vi "Test TCC Request Chamber State Returns Heater State.vi"(8 "error in (no error)":errorcluster, 11 "Thermal Chamber Controller Test In":refnum<class "Thermal Chamber Controller Test.lvclass">) -> (0 "error out":errorcluster, 3 "Thermal Chamber Controller Test Out":refnum<class "Thermal Chamber Controller Test.lvclass">)   [LabVIEW 2020, in "Thermal Chamber Controller Test.lvclass"]
uses:
  Thermal Chamber Controller Test.lvclass
  C:/Program Files (x86)/National Instruments/LabVIEW 2020/vi.lib/Astemes/LUnit/Test Case.lvclass
  Thermal Chamber Controller/Thermal Chamber Controller.lvclass
  C:/Program Files (x86)/National Instruments/LabVIEW 2020/vi.lib/Astemes/Triarc Framework/Process/Process.lvclass
  Thermal Chamber Controller/Private/Heater State.ctl
  <vilib>/Astemes/Triarc Framework/Process/Process.lvclass/Process.ctl
  <vilib>/Astemes/LUnit/Test Case.lvclass/Test Case.ctl
  <vilib>/Astemes/Triarc Framework/Process/Private/SubVIs/Wait for finish.vi
  <vilib>/Astemes/Triarc Framework/Process/Private/SubVIs/Set Lifecycle State.vi
  <vilib>/Astemes/Triarc Framework/Process/Protected/Messaging/Send Message.vi
  <vilib>/Astemes/Triarc Framework/Process/Public/Lifecycle/Get Lifecycle State.vi
  <vilib>/Astemes/LUnit/Palette/Fail.vi
  <vilib>/Astemes/LUnit/Palette/Pass.vi
  <vilib>/Astemes/LUnit/Set Assertion Type.vi
  <vilib>/Astemes/Triarc Framework/Process/Private/SubVIs/Handle Debug Data.vi
  <vilib>/Utility/error.llb/Clear Errors.vi
  <vilib>/Astemes/LUnit/Add test result.vi
  <vilib>/Utility/High Resolution Relative Seconds.vi
  <vilib>/Astemes/LUnit/LUnit Record Assertion Result.vi
  <vilib>/Astemes/LUnit/LUnit Aggregate Assertion Results.vi
  <vilib>/Astemes/LUnit/Method Result/LUnit Merge Status.vi
  <vilib>/Astemes/LUnit/LUnit Concatenate result strings.vi
  <vilib>/Utility/error.llb/Error Cluster From Error Code.vi
  <vilib>/Astemes/Triarc Framework/Process/Process.lvclass
  <vilib>/Astemes/LUnit/Test Case.lvclass
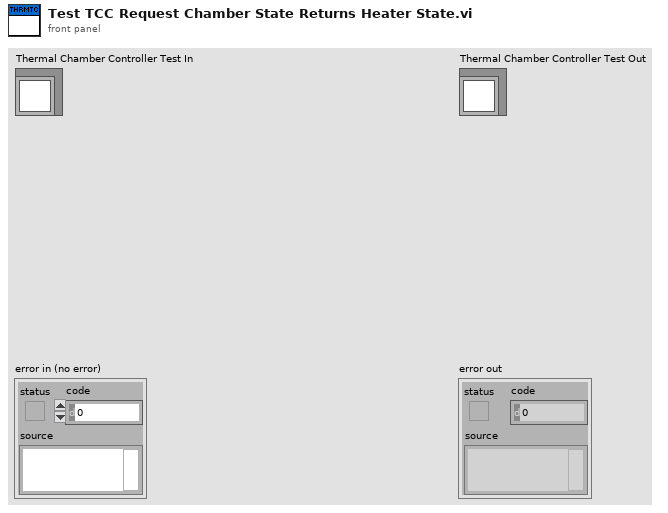
[diagram p1: front panel]
types:
  T1 = typedef "Thermal Chamber Controller.lvclass/Heater State.ctl" = enum16{"Heater Disabled", "Heater Enabled"}
  T2 = typedef "Thermal Chamber Controller.lvclass/Chamber State.ctl" = cluster{"Actual Temperature":dbl, "Temperature Set Point":dbl, "Temperature Ramp Rate":dbl, "Heater State":T1}
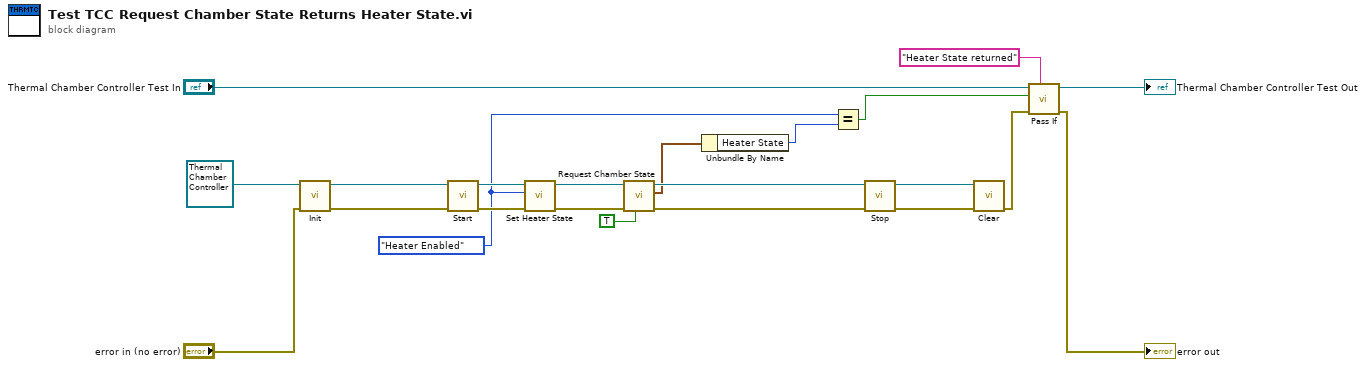
[diagram p0: block diagram]
diagram:
  w3 = Heater_State."Heater Enabled" ("Heater State")
  n1 = call-dynamic "Init.vi"("error in (no error)"="error in (no error)", "View In"=refnum<class "Thermal Chamber Controller.lvclass"> refnum ("Thermal Chamber Controller.lvclass")) -> ("error out"=w16:errorcluster, "View Out"=w17:refnum<class "Thermal Chamber Controller.lvclass">)  [unwired: 8 in]
  n2 = call <vilib>:"Start.vi"("error in (no error)"=w16, "Process In"=w17) -> ("error out"=w21:errorcluster, "Process Out"=w9:refnum<class "Thermal Chamber Controller.lvclass">)  [unwired: 7 in, 1 out]
  n3 = call "Set Heater State.vi"("error in (no error)"=w21, "Heater State"=w3, "Thermal Chamber Controller In"=w9) -> ("error out"=w10:errorcluster, "Thermal Chamber Controller Out"=w8:refnum<class "Thermal Chamber Controller.lvclass">)  [unwired: 7 in]
  n4 = call "Request Chamber State.vi"("wait for reply (T)"=TRUE, "error in (no error)"=w10, "Thermal Chamber Controller In"=w8) -> ("error out"=w15:errorcluster, "Chamber Status Reply Payload"=w11:T2, "Thermal Chamber Controller Out"=w20:refnum<class "Thermal Chamber Controller.lvclass">)  [unwired: 5 in, 1 out]
  n5 = Unbundle By Name(w11) -> ("Heater State"=w2:T1)
  n6 = Equal?(x=w3, y=w2) -> (x = y?=w1:bool)
  n7 = call <vilib>:"Stop.vi"("error in (no error)"=w15, "Process In"=w20) -> ("error out"=w18:errorcluster, "Process Out"=w19:refnum<class "Thermal Chamber Controller.lvclass">)  [unwired: 7 in, 1 out]
  n8 = call-dynamic "Clear.vi"("error in (no error)"=w18, "View In"=w19) -> ("error out"=w6:errorcluster)  [unwired: 9 in]
  n9 = call <vilib>:"Pass If.vi"("Description"="Heater State returned", "error in (no error)"=w6, "Pass?"=w1, "LUnit Test Case In"="Thermal Chamber Controller Test In") -> ("error out"=→"error out":errorcluster, "LUnit Test Case Out"=→"Thermal Chamber Controller Test Out":refnum<class "Thermal Chamber Controller Test.lvclass">)  [unwired: 6 in]
